vi "Config sinus penta.vi"(11 "stato config":T1) -> ()   [LabVIEW 2019]
uses:
  SINUS PENTA SANTERNO/controls/Dati targa sinus penta.ctl
panel:
  in  "Cancel Button":bool
  in  "OK Button":bool
  in  "DATI TARGA sinus penta":T2 {"Freq nominale del motore Mot1" format="%.1f"; "Potenza nominale del motore Mot1" format="%.1f"; "Corrente nominale del motore Mot1" format="%.1f"; "Tensione nominale del motore mot1" format="%.1f"}
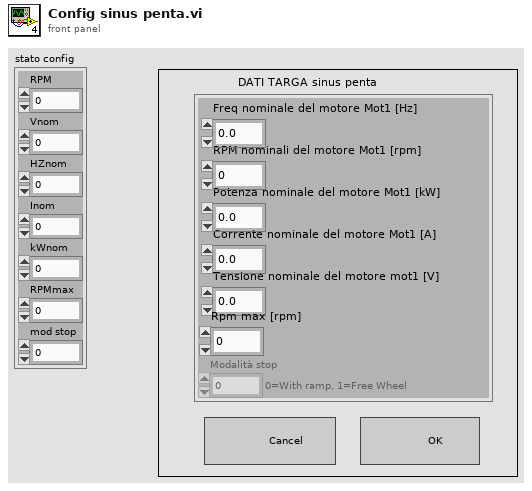
[diagram p1: front panel]
types:
  T1 = cluster{"RPM":dbl, "Vnom":dbl, "HZnom":dbl, "Inom":dbl, "kWnom":dbl, "RPMmax":dbl, "mod stop":dbl}
  T2 = typedef "Dati targa sinus penta.ctl" = cluster{"Freq nominale del motore Mot1":dbl, "RPM nominali del motore Mot1":i16, "Potenza nominale del motore Mot1":dbl, "Corrente nominale del motore Mot1":dbl, "Tensione nominale del motore mot1":dbl, "Rpm max":u16, "Modalità stop":u16}
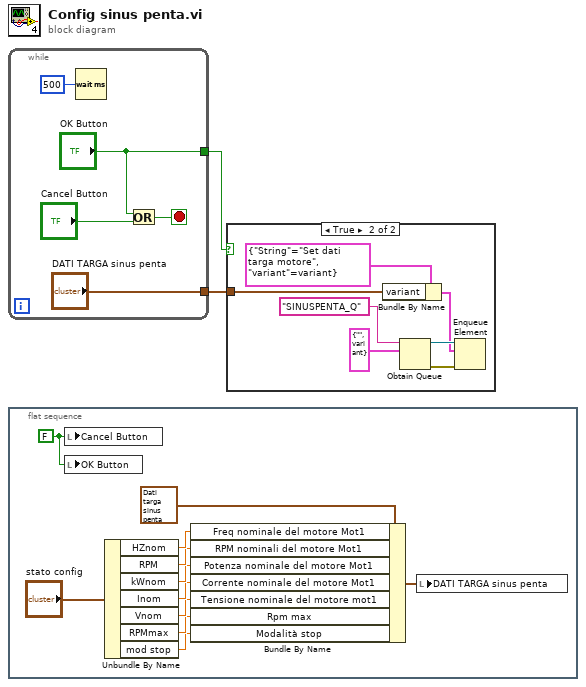
[diagram p0: block diagram]
diagram:
  n1 = while {
    tunnel: ["OK Button"] -> w2
    tunnel: ["DATI TARGA sinus penta"] -> w1
    stop <- w6 stop-if-true
    n2 = Wait (ms)(milliseconds to wait=u32 500) -> ()  [unwired: 1 out]
    n3 = Or(x="OK Button", y="Cancel Button") -> (x .or. y?=w6:bool)
  }
  n4 = flat-sequence {
    frame #0 {
      w18 = FALSE ("Cancel Button")
      n5 = local write "Cancel Button"(w18) -> ()
      n6 = local write "OK Button"(w18) -> ()
      n7 = Unbundle By Name("stato config") -> ("HZnom"=w15:dbl, "RPM"=w14:dbl, "kWnom"=w13:dbl, "Inom"=w12:dbl, "Vnom"=w11:dbl, "RPMmax"=w10:dbl, "mod stop"=w9:dbl)
      n8 = Bundle By Name(cluster=T2 {"Freq nominale del motore Mot1"=50.0, "RPM nominali del motore Mot1"=2950, "Potenza nominale del motore Mot1"=12.0, "Corrente nominale del motore Mot1"=24.0, "Tensione nominale del motore mot1"=400.0, "Rpm max"=3000, "Modalità stop"=0} ("DATI TARGA sinus penta"), "Freq nominale del motore Mot1"=w15, "RPM nominali del motore Mot1"=w14, "Potenza nominale del motore Mot1"=w13, "Corrente nominale del motore Mot1"=w12, "Tensione nominale del motore mot1"=w11, "Rpm max"=w10, "Modalità stop"=w9) -> (w16:T2)
      n9 = local write "DATI TARGA sinus penta"(w16) -> ()
    }
  }
  n10 = case shown="True" w2 {
    tunnel: w1 -> [_ w19]
    frame False {
    }
    frame True {
      n11 = Bundle By Name(cluster=cluster{"String":string, "variant":variant} {"String"="Set dati targa motore", "variant"=variant} ("element"), "variant"=w19) -> (w20:cluster{"String":string, "variant":variant})
      n12 = Obtain Queue(name (unnamed)="SINUSPENTA_Q", element data type=cluster{"String":string, "variant":variant} {"String"="", "variant"=variant} ("element")) -> (queue out=w22:refnum<queue>, error out=w24:errorcluster)  [unwired: 3 in, 1 out]
      n13 = Enqueue Element(queue=w22, element=w20, error in (no error)=w24) -> ()  [unwired: 1 in, 3 out]
    }
  }
